vi "rs3 capture single 2.vi"(0 "queue in":u64, 5 "timeout":u32=5000, 11 "error in (no error)":errorcluster) -> (1 "Capture Error":string="No Error", 2 "Frame number":u64, 3 "RS Format":u16(ring)=6 items=["    RS2_FORMAT_ANY             , /**< When passed to enable stream, librealsense will try to provide best suited format */", "    RS2_FORMAT_Z16             , /**< 16-bit linear depth values. The depth is meters is equal to depth scale * pixel value. */", "    RS2_FORMAT_DISPARITY16     , /**< 16-bit linear disparity values. The depth in meters is equal to depth scale / pixel value. */", "    RS2_FORMAT_XYZ32F          , /**< 32-bit floating point 3D coordinates. */", "    RS2_FORMAT_YUYV            , /**< Standard YUV pixel format as described in https://en.wikipedia.org/wiki/YUV */", "    RS2_FORMAT_RGB8            , /**< 8-bit red, green and blue channels */", "    RS2_FORMAT_BGR8            , /**< 8-bit blue, green, and red channels -- suitable for OpenCV */", "    RS2_FORMAT_RGBA8           , /**< 8-bit red, green and blue channels + constant alpha channel equal to FF */", "    RS2_FORMAT_BGRA8           , /**< 8-bit blue, green, and red channels + constant alpha channel equal to FF */", "    RS2_FORMAT_Y8              , /**< 8-bit per-pixel grayscale image */", "    RS2_FORMAT_Y16             , /**< 16-bit per-pixel grayscale image */", "    RS2_FORMAT_RAW10           , /**< Four 10-bit luminance values encoded into a 5-byte macropixel */", "    RS2_FORMAT_RAW16           , /**< 16-bit raw image */", "    RS2_FORMAT_RAW8            , /**< 8-bit raw image */", "    RS2_FORMAT_UYVY            , /**< Similar to the standard YUYV pixel format, but packed in a different order */", "    RS2_FORMAT_MOTION_RAW      , /**< Raw data from the motion sensor */", "    RS2_FORMAT_MOTION_XYZ32F   , /**< Motion data packed as 3 32-bit float values, for X, Y, and Z axis */", "    RS2_FORMAT_GPIO_RAW        , /**< Raw data from the external sensors hooked to one of the GPIO's */", "    RS2_FORMAT_COUNT             /**< Number of enumeration values. Not a valid input: intended to be used in for-loops. */"], 4 "RS Stream":u16(ring) items=["    RS2_STREAM_ANY,", "    RS2_STREAM_DEPTH                            , /**< Native stream of depth data produced by RealSense device */", "    RS2_STREAM_COLOR                            , /**< Native stream of color data captured by RealSense device */", "    RS2_STREAM_INFRARED                         , /**< Native stream of infrared data captured by RealSense device */", "    RS2_STREAM_FISHEYE                          , /**< Native stream of fish-eye (wide) data captured from the dedicate motion camera */", "    RS2_STREAM_GYRO                             , /**< Native stream of gyroscope motion data produced by RealSense device */", "    RS2_STREAM_ACCEL                            , /**< Native stream of accelerometer motion data produced by RealSense device */", "    RS2_STREAM_GPIO                             , /**< Signals from external device connected through GPIO */", "    RS2_STREAM_COUNT"], 6 "frame out":u64, 8 "width":i32, 10 "Stream type":T1(ring), 12 "index":i32, 13 "Time stamp":dbl, 14 "height":i32, 15 "error out":errorcluster)   [LabVIEW 2017, in "libRealSense3.lvlib"]
doc: "This VI waits for and returns the FRAME handle of captured data. \nIt also queries the frame profile to identify the type of stream data it was. \nThis type is output into the \"Stream Type\":\n\n0 Depth\n3 Color left\n5 IR Left \n9 IR Right\n21 IR Left (Y16)\n25 IR RIght (Y16)"
uses:
  <vilib>/addons/RealSense/libRealSense3.lvlib
panel:
  # "RS3 Capture Single 2"
  # "(C) Intel Corp. 2017,  AGJ"
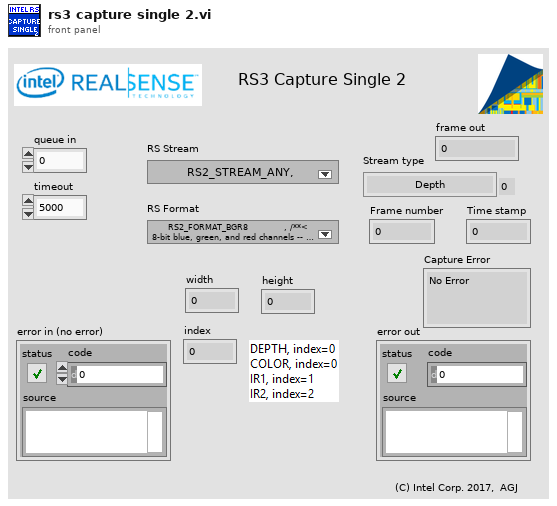
[diagram p1: front panel]
types:
  T1 = enum16{"Depth", "Color (ext.)", "Color (left) ", "IR Left", "IR Right", "IR Left (Y16)", "IR Right (Y16)"}
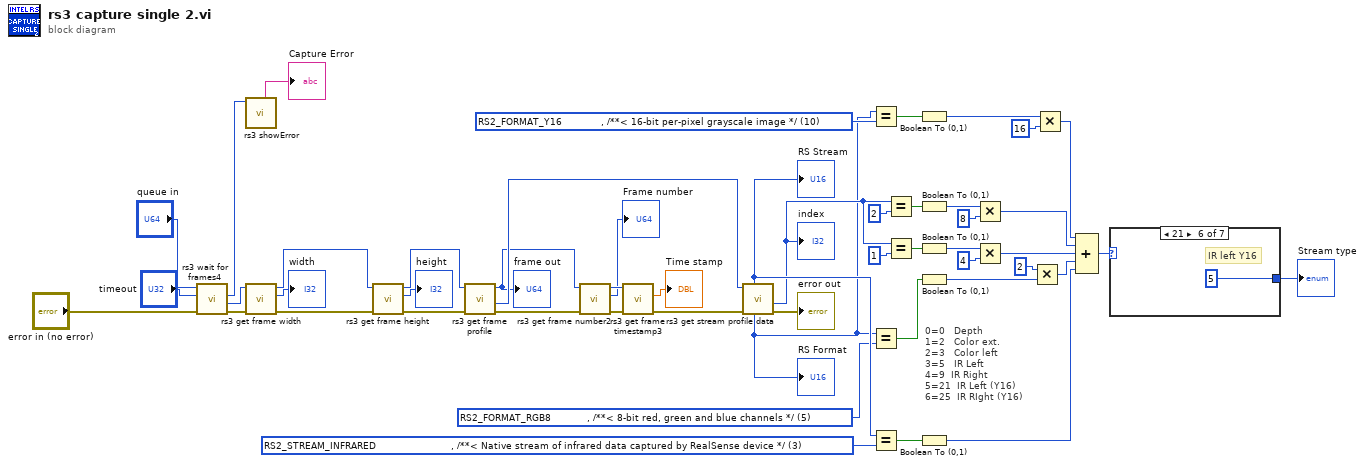
[diagram p0: block diagram]
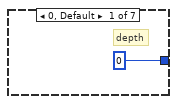
[diagram p2: hidden frame]
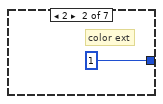
[diagram p3: hidden frame]
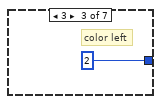
[diagram p4: hidden frame]
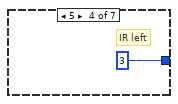
[diagram p5: hidden frame]
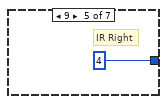
[diagram p6: hidden frame]
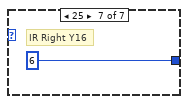
[diagram p7: hidden frame]
diagram:
  w13 = u16 10 items=["    RS2_FORMAT_ANY             , /**< When passed to enable stream, librealsense will try to provide best suited format */", "    RS2_FORMAT_Z16             , /**< 16-bit linear depth values. The depth is meters is equal to depth scale * pixel value. */", "    RS2_FORMAT_DISPARITY16     , /**< 16-bit linear disparity values. The depth in meters is equal to depth scale / pixel value. */", "    RS2_FORMAT_XYZ32F          , /**< 32-bit floating point 3D coordinates. */", "    RS2_FORMAT_YUYV            , /**< Standard YUV pixel format as described in https://en.wikipedia.org/wiki/YUV */", "    RS2_FORMAT_RGB8            , /**< 8-bit red, green and blue channels */", "    RS2_FORMAT_BGR8            , /**< 8-bit blue, green, and red channels -- suitable for OpenCV */", "    RS2_FORMAT_RGBA8           , /**< 8-bit red, green and blue channels + constant alpha channel equal to FF */", "    RS2_FORMAT_BGRA8           , /**< 8-bit blue, green, and red channels + constant alpha channel equal to FF */", "    RS2_FORMAT_Y8              , /**< 8-bit per-pixel grayscale image */", "    RS2_FORMAT_Y16             , /**< 16-bit per-pixel grayscale image */", "    RS2_FORMAT_RAW10           , /**< Four 10-bit luminance values encoded into a 5-byte macropixel */", "    RS2_FORMAT_RAW16           , /**< 16-bit raw image */", "    RS2_FORMAT_RAW8            , /**< 8-bit raw image */", "    RS2_FORMAT_UYVY            , /**< Similar to the standard YUYV pixel format, but packed in a different order */", "    RS2_FORMAT_MOTION_RAW      , /**< Raw data from the motion sensor */", "    RS2_FORMAT_MOTION_XYZ32F   , /**< Motion data packed as 3 32-bit float values, for X, Y, and Z axis */", "    RS2_FORMAT_GPIO_RAW        , /**< Raw data from the external sensors hooked to one of the GPIO's */", "    RS2_FORMAT_COUNT             /**< Number of enumeration values. Not a valid input: intended to be used in for-loops. */"] ("RS Format")
  w35 = u16 3 items=["    RS2_STREAM_ANY,", "    RS2_STREAM_DEPTH                            , /**< Native stream of depth data produced by RealSense device */", "    RS2_STREAM_COLOR                            , /**< Native stream of color data captured by RealSense device */", "    RS2_STREAM_INFRARED                         , /**< Native stream of infrared data captured by RealSense device */", "    RS2_STREAM_FISHEYE                          , /**< Native stream of fish-eye (wide) data captured from the dedicate motion camera */", "    RS2_STREAM_GYRO                             , /**< Native stream of gyroscope motion data produced by RealSense device */", "    RS2_STREAM_ACCEL                            , /**< Native stream of accelerometer motion data produced by RealSense device */", "    RS2_STREAM_GPIO                             , /**< Signals from external device connected through GPIO */", "    RS2_STREAM_COUNT"] ("RS Stream")
  w12 = u16 5 items=["    RS2_FORMAT_ANY             , /**< When passed to enable stream, librealsense will try to provide best suited format */", "    RS2_FORMAT_Z16             , /**< 16-bit linear depth values. The depth is meters is equal to depth scale * pixel value. */", "    RS2_FORMAT_DISPARITY16     , /**< 16-bit linear disparity values. The depth in meters is equal to depth scale / pixel value. */", "    RS2_FORMAT_XYZ32F          , /**< 32-bit floating point 3D coordinates. */", "    RS2_FORMAT_YUYV            , /**< Standard YUV pixel format as described in https://en.wikipedia.org/wiki/YUV */", "    RS2_FORMAT_RGB8            , /**< 8-bit red, green and blue channels */", "    RS2_FORMAT_BGR8            , /**< 8-bit blue, green, and red channels -- suitable for OpenCV */", "    RS2_FORMAT_RGBA8           , /**< 8-bit red, green and blue channels + constant alpha channel equal to FF */", "    RS2_FORMAT_BGRA8           , /**< 8-bit blue, green, and red channels + constant alpha channel equal to FF */", "    RS2_FORMAT_Y8              , /**< 8-bit per-pixel grayscale image */", "    RS2_FORMAT_Y16             , /**< 16-bit per-pixel grayscale image */", "    RS2_FORMAT_RAW10           , /**< Four 10-bit luminance values encoded into a 5-byte macropixel */", "    RS2_FORMAT_RAW16           , /**< 16-bit raw image */", "    RS2_FORMAT_RAW8            , /**< 8-bit raw image */", "    RS2_FORMAT_UYVY            , /**< Similar to the standard YUYV pixel format, but packed in a different order */", "    RS2_FORMAT_MOTION_RAW      , /**< Raw data from the motion sensor */", "    RS2_FORMAT_MOTION_XYZ32F   , /**< Motion data packed as 3 32-bit float values, for X, Y, and Z axis */", "    RS2_FORMAT_GPIO_RAW        , /**< Raw data from the external sensors hooked to one of the GPIO's */", "    RS2_FORMAT_COUNT             /**< Number of enumeration values. Not a valid input: intended to be used in for-loops. */"] ("RS Format")
  # "0=0   Depth\n1=2   Color ext.\n2=3   Color left\n3=5   IR Left \n4=9  IR Right\n5=21  IR Left (Y16)\n6=25  IR RIght (Y16)"
  n1 = call <vilib>:"rs3 wait for frames4.vi"("error in (no error)"="error in (no error)", 10:"timeout", 11:"queue in") -> (0:"error out"=w42:errorcluster, "frame"=w48:u64, 2:"error out"=w39:u64)  [unwired: 6 in]
  n2 = call <vilib>:"rs3 showError.vi"("error"=w39) -> ("Error summary"=→"Capture Error":string)  [unwired: 6 in, 4 out]
  n3 = call <vilib>:"rs3 get frame width.vi"("error in (no error)"=w42, "frame in"=w48) -> ("error out"=w41:errorcluster, "width"=→"width":i32, "Frame out"=w46:u64)  [unwired: 6 in, 1 out]
  n4 = call <vilib>:"rs3 get frame height.vi"("error in (no error)"=w41, "frame in"=w46) -> ("error out"=w43:errorcluster, "height"=→"height":i32, "Frame out"=w47:u64)  [unwired: 6 in, 1 out]
  n5 = call <vilib>:"rs3 get frame profile.vi"("error in (no error)"=w43, "Frame"=w47) -> ("error out"=w5:errorcluster, "stream profile"=w40:u64, "frame out"=w9:u64)  [unwired: 6 in, 1 out]
  "frame out" <- w9
  n6 = call <vilib>:"rs3 get frame number2.vi"("error in (no error)"=w5, "frame in"=w9) -> ("error out"=w4:errorcluster, "Frame number"=→"Frame number":u64, "frame out"=w8:u64)  [unwired: 6 in, 1 out]
  n7 = call <vilib>:"rs3 get frame timestamp3.vi"("error in (no error)"=w4, "frame in"=w8) -> ("error out"=w3:errorcluster, "Time stamp"=→"Time stamp":dbl)  [unwired: 6 in, 2 out]
  n8 = call <vilib>:"rs3 get stream profile data.vi"("error in (no error)"=w3, "Profile"=w40) -> ("error out"=→"error out":errorcluster, "index"=w18:i32, "RS Format"=w10:u16, "RS Stream"=w34:u16)  [unwired: 2 in, 4 out]
  "RS Format" <- w10
  "RS Stream" <- w34
  "index" <- w18
  n9 = Equal?(x=w10, y=w13) -> (x = y?=w14:bool)
  n10 = Equal?(x=w10, y=w12) -> (x = y?=w31:bool)
  n11 = Equal?(x=w34, y=w35) -> (x = y?=w30:bool)
  n12 = Equal?(x=w18, y=2) -> (x = y?=w20:bool)
  n13 = Equal?(x=w18, y=1) -> (x = y?=w32:bool)
  n14 = Boolean To (0,1)(Boolean=w14) -> (0, 1=w16:i16)
  n15 = Boolean To (0,1)(Boolean=w20) -> (0, 1=w21:i16)
  n16 = Boolean To (0,1)(Boolean=w32) -> (0, 1=w27:i16)
  n17 = Boolean To (0,1)(Boolean=w31) -> (0, 1=w29:i16)
  n18 = Boolean To (0,1)(Boolean=w30) -> (0, 1=w24:i16)
  n19 = Multiply(x=w21, y=i16 8) -> (x*y=w17:i16)
  n20 = Multiply(x=w27, y=i16 4) -> (x*y=w23:i16)
  n21 = Multiply(x=i16 2, y=w29) -> (x*y=w25:i16)
  n22 = Multiply(x=w16, y=i16 16) -> (x*y=w11:i16)
  n23 = Compound Arithmetic op=ADD(w11, w17, w23, w25, w24) -> (w2:i16)
  n24 = case shown="21" w2 {
    tunnel: [0 1 2 3 4 5 6] -> w1
    frame 0, Default {
      # "depth"
    }
    frame 2 {
      # "color ext"
    }
    frame 3 {
      # "color left"
    }
    frame 5 {
      # "IR left"
    }
    frame 9 {
      # "IR Right"
    }
    frame 21 {
      # "IR left Y16"
    }
    frame 25 {
      # "IR Right Y16"
    }
  }
  "Stream type" <- w1
